vi "relative access path.vi"(11 "Oauth2.QBO":refnum<class "Oauth2.QBO.lvclass">) -> (1 "Token Access Path":string, 2 "Authorization Path":string)   [LabVIEW 2013, in "Oauth2.QBO.lvclass"]
uses:
  Oauth2.QBO.lvclass
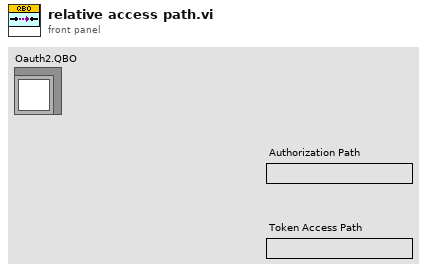
[diagram p1: front panel]
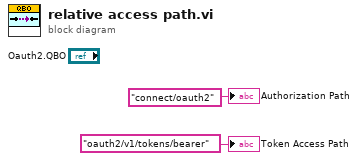
[diagram p0: block diagram]
diagram:
  "Authorization Path" <- "connect/oauth2" ("Authorization Path")
  "Token Access Path" <- "oauth2/v1/tokens/bearer" ("Authorization Path")
